vi "ABR-Compute Final Average.vi"(0 "#Avgs":i32, 1 "Remove DC Offset":bool=TRUE, 5 "Running Sum 1":dbl[](array[numeric]), 9 "Running Sum 2":dbl[](array[numeric]), 11 "AltPol":bool, 12 "Avg Mode":enum16{"Neural/CM", "ANOW"}(ring)) -> (6 "Neural":dbl[](array[numeric]), 10 "Microphonic":dbl[](array[numeric]))   [LabVIEW 2020]
uses:
  <vilib>/Analysis/baseanly.llb/Mean (DBL).vi
  <vilib>/Analysis/NI_AALBase.lvlib
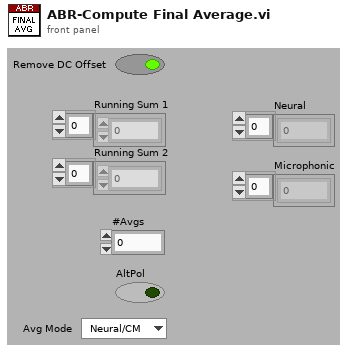
[diagram p1: front panel]
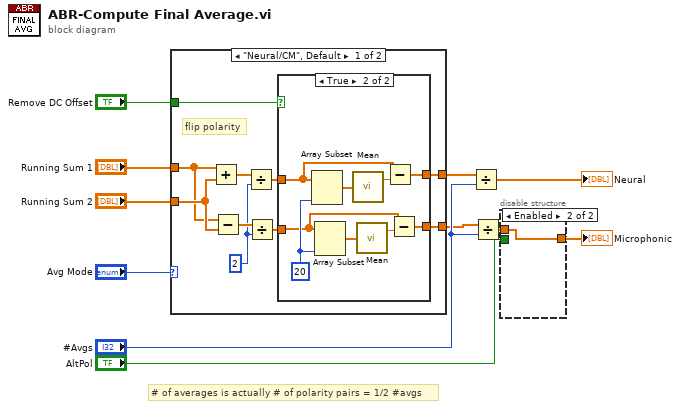
[diagram p0: block diagram]
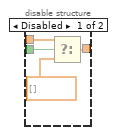
[diagram p2: hidden frame]
diagram:
  # "# of averages is actually # of polarity pairs = 1/2 #avgs"
  n1 = case shown="\"Neural/CM\", Default" "Avg Mode" {
    tunnel: "Remove DC Offset" -> [w20 _]
    tunnel: [w18 w33] -> w5
    tunnel: [w17 w34] -> w4
    tunnel: "Running Sum 2" -> [w16 w33]
    tunnel: "Running Sum 1" -> [w15 w34]
    frame "Neural/CM", Default {
      w12 = 2
      # "flip polarity"
      n2 = Add(x=w15, y=w16) -> (x+y=w21:dbl[])
      n3 = Subtract(x=w15, y=w16) -> (x-y=w19:dbl[])
      n4 = Divide(x=w21, y=w12) -> (x/y=w14:dbl[])
      n5 = Divide(x=w19, y=w12) -> (x/y=w13:dbl[])
      n6 = case shown="True" w20 {
        tunnel: [w23 w27] -> w17
        tunnel: w14 -> [w23 w28]
        tunnel: [w22 w24] -> w18
        tunnel: w13 -> [w22 w26]
        frame False {
        }
        frame True {
          w32 = 20
          n7 = Array Subset(array=w28, length=w32) -> (w30:dbl[])  [unwired: 1 in]
          n8 = Array Subset(array=w26, length=w32) -> (w31:dbl[])  [unwired: 1 in]
          n9 = call-poly <vilib>:"Mean.vi"("X"=w30) -> ("mean"=w29:dbl)  [unwired: 1 out]
          n10 = call-poly <vilib>:"Mean.vi"("X"=w31) -> ("mean"=w25:dbl)  [unwired: 1 out]
          n11 = Subtract(x=w28, y=w29) -> (x-y=w27:dbl[])
          n12 = Subtract(x=w26, y=w25) -> (x-y=w24:dbl[])
        }
      }
    }
    frame "ANOW" {
    }
  }
  n13 = Divide(x=w4, y="#Avgs") -> (x/y=→"Neural":dbl[])
  n14 = Divide(x=w5, y="#Avgs") -> (x/y=w7:dbl[])
  n15 = disable-structure shown="Enabled" {
    disable-tunnel: "AltPol" -> [w38 _]
    disable-tunnel: [w36 w39] -> w8
    disable-tunnel: w7 -> [w35 w39]
    frame Disabled {
      n16 = Select(t=w35, s=w38, f=ext[] []) -> (s? t:f=w36:ext[])
    }
    frame Enabled {
    }
  }
  "Microphonic" <- w8
